vi "Delay without Error Handling.vi"(8 "error in (no error)":errorcluster, 9 "Delay (ms)":u32) -> (0 "error out":errorcluster)   [LabVIEW 2018, in "Utilities.lvlib"]
uses:
  Utilities.lvlib
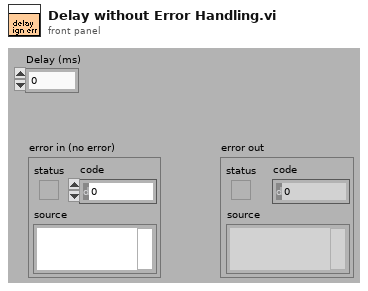
[diagram p1: front panel]
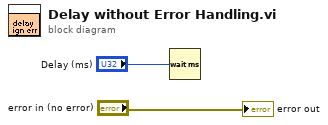
[diagram p0: block diagram]
diagram:
  n1 = Wait (ms)(milliseconds to wait="Delay (ms)") -> ()  [unwired: 1 out]
  "error out" <- "error in (no error)"
